vi "Build Shared Library Search Path.vi"(8 "Error In":errorcluster, 11 "labssh2 Shared Library":path=path "") -> (0 "Error Out":errorcluster, 3 "Search Path":path[](array[path])=[path "D:/Users/cfield/Code/Field R&D Services/SSH/LabSSH2/LabVIEW/trunk/src/LabSSH2/Private/labssh2.*"])   [LabVIEW 2017, in "Toolkit.lvlib"]
uses:
  Toolkit.lvlib
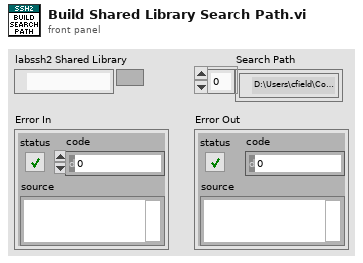
[diagram p1: front panel]
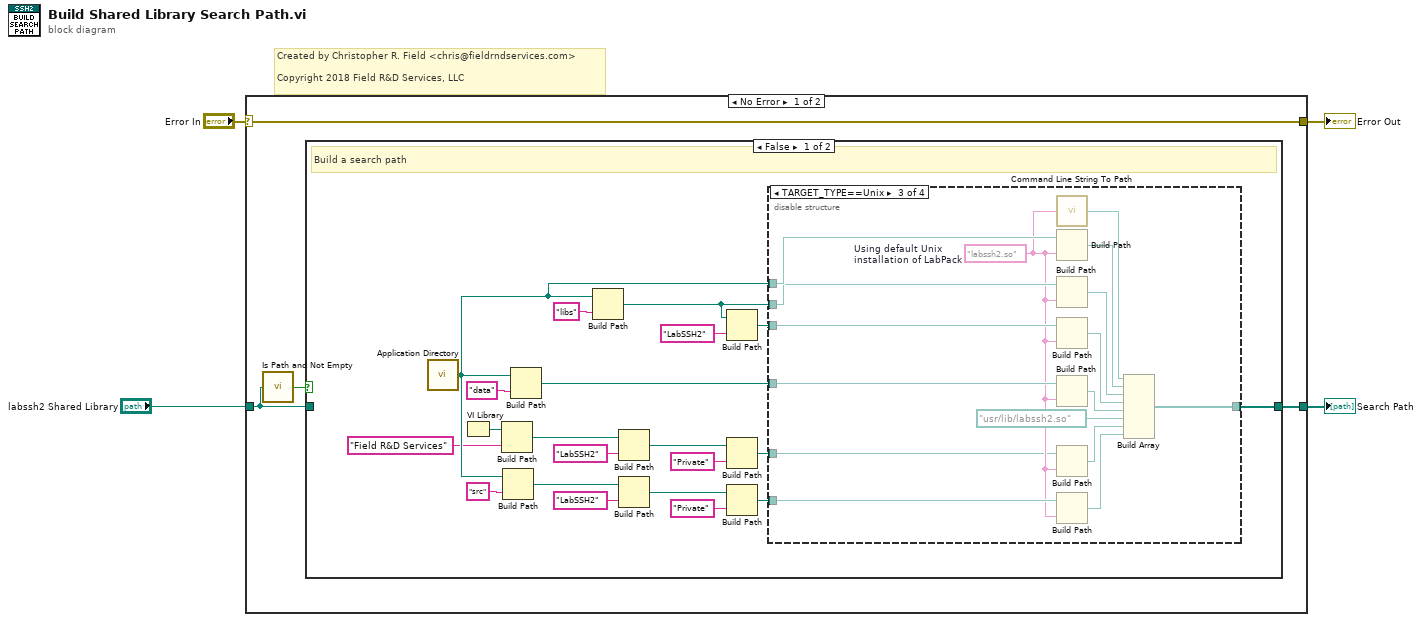
[diagram p0: block diagram]
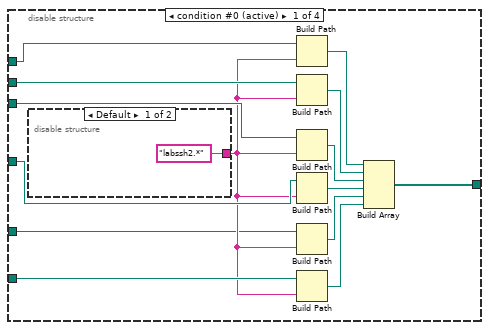
[diagram p2: hidden frame]
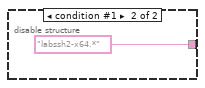
[diagram p3: hidden frame]
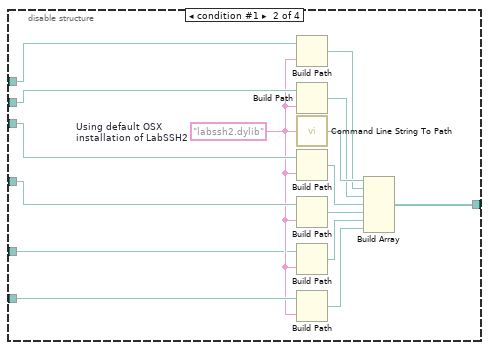
[diagram p4: hidden frame]
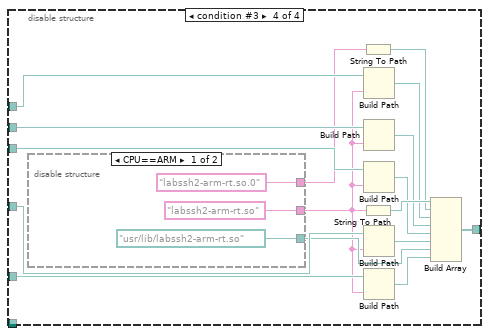
[diagram p5: hidden frame]
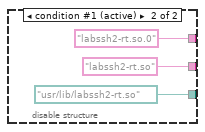
[diagram p6: hidden frame]
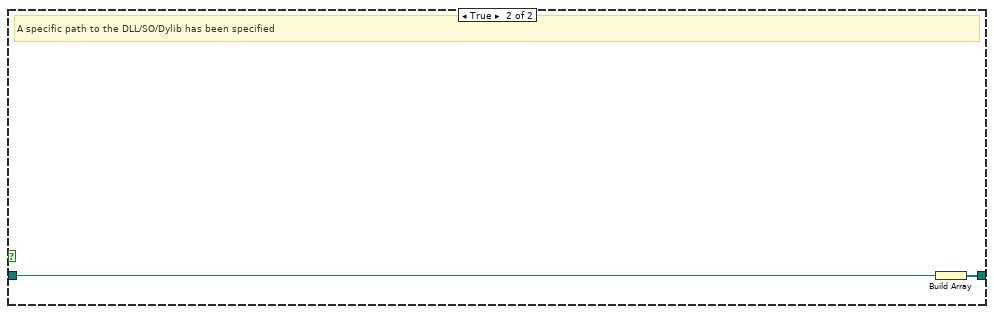
[diagram p7: hidden frame]
diagram:
  # "Created by Christopher R. Field <chris@fieldrndservices.com>\n\nCopyright 2018 Field R&D Services, LLC"
  n1 = case shown="No Error" "Error In" {
    selector: "Error In" -> [w5 w101]
    tunnel: [w8 _] -> w4
    tunnel: "labssh2 Shared Library" -> [w7 _]
    tunnel: [w5 w101] -> w1
    frame No Error {
      n2 = call <vilib>:"Is Path and Not Empty.vi"("path"=w7) -> ("Is Path and Not Empty?"=w6:bool)  [unwired: 4 in]
      n3 = case shown="False" w6 {
        tunnel: w7 -> [_ w100]
        tunnel: [w23 w99] -> w8
        frame False {
          # "Build a search path"
          n4 = call <vilib>:"Application Directory.vi"() -> ("Application Directory"=w21:path)
          n5 = VI Library() -> (path=w15:path)
          n6 = Build Path(base path=w15, name or relative path="Field R&D Services") -> (appended path=w13:path)
          n7 = Build Path ("EXE include\nlocation")(base path=w21, name or relative path="src") -> (appended path=w26:path)
          n8 = Build Path ("EXE include\nlocation")(base path=w21, name or relative path="data") -> (appended path=w19:path)
          n9 = Build Path ("EXE include\nlocation")(base path=w21, name or relative path="libs") -> (appended path=w18:path)
          n10 = Build Path(base path=w13, name or relative path="LabSSH2") -> (appended path=w11:path)
          n11 = Build Path ("EXE include\nlocation")(base path=w26, name or relative path="LabSSH2") -> (appended path=w28:path)
          n12 = Build Path ("EXE include\nlocation")(base path=w18, name or relative path="LabSSH2") -> (appended path=w16:path)
          n13 = Build Path(base path=w11, name or relative path="Private") -> (appended path=w9:path)
          n14 = Build Path ("EXE include\nlocation")(base path=w28, name or relative path="Private") -> (appended path=w24:path)
          n15 = disable-structure shown="TARGET_TYPE==Unix" {
            disable-tunnel: [w42 w59 w75 w92] -> w23
            disable-tunnel: w24 -> [w43 w58 w74 _]
            disable-tunnel: w21 -> [w41 w57 w68 w85]
            disable-tunnel: w18 -> [w40 w56 w67 w84]
            disable-tunnel: w19 -> [w39 w54 w65 w82]
            disable-tunnel: w16 -> [w38 w55 w66 w83]
            disable-tunnel: w9 -> [w36 w48 w63 w79]
            frame condition #0 (active) {
              n16 = disable-structure shown="Default" {
                disable-tunnel: ["labssh2.*" ("name or relative path") "labssh2-x64.*" ("name or relative path")] -> w37
                frame condition #0 (active) {
                }
                frame condition #1 {
                }
              }
              n17 = Build Path ("EXE include\nlocation")(base path=w41, name or relative path=w37) -> (appended path=w30:path)
              n18 = Build Path ("EXE include\nlocation")(base path=w40, name or relative path=w37) -> (appended path=w31:path)
              n19 = Build Path ("EXE include\nlocation")(base path=w38, name or relative path=w37) -> (appended path=w32:path)
              n20 = Build Path ("EXE include\nlocation")(base path=w39, name or relative path=w37) -> (appended path=w33:path)
              n21 = Build Path ("EXE include\nlocation")(base path=w36, name or relative path=w37) -> (appended path=w35:path)
              n22 = Build Path ("EXE include\nlocation")(base path=w43, name or relative path=w37) -> (appended path=w34:path)
              n23 = Build Array(w30, w31, w32, w33, w35, w34) -> (w42:path[])
            }
            frame condition #1 {
              w49 = "labssh2.dylib"  # Using default OSX installation of LabSSH2
              n24 = Build Path ("EXE include\nlocation")(base path=w57, name or relative path=w49) -> (appended path=w53:path)
              n25 = Build Path ("EXE include\nlocation")(base path=w56, name or relative path=w49) -> (appended path=w52:path)
              n26 = call <vilib>:"Command Line String To Path.vi"("string"=w49) -> ("path"=w60:path)
              n27 = Build Path ("EXE include\nlocation")(base path=w55, name or relative path=w49) -> (appended path=w51:path)
              n28 = Build Path ("EXE include\nlocation")(base path=w54, name or relative path=w49) -> (appended path=w50:path)
              n29 = Build Path ("EXE include\nlocation")(base path=w48, name or relative path=w49) -> (appended path=w47:path)
              n30 = Build Path ("EXE include\nlocation")(base path=w58, name or relative path=w49) -> (appended path=w46:path)
              n31 = Build Array(w60, w53, w52, w51, w50, w47, w46) -> (w59:path[])
            }
            frame condition #2 {
              w64 = "labssh2.so"  # Using default Unix installation of LabPack
              n32 = call <vilib>:"Command Line String To Path.vi"("string"=w64) -> ("path"=w76:path)
              n33 = Build Path ("EXE include\nlocation")(base path=w68, name or relative path=w64) -> (appended path=w72:path)
              n34 = Build Path ("EXE include\nlocation")(base path=w67, name or relative path=w64) -> (appended path=w71:path)
              n35 = Build Path ("EXE include\nlocation")(base path=w66, name or relative path=w64) -> (appended path=w70:path)
              n36 = Build Path ("EXE include\nlocation")(base path=w65, name or relative path=w64) -> (appended path=w69:path)
              n37 = Build Path ("EXE include\nlocation")(base path=w63, name or relative path=w64) -> (appended path=w62:path)
              n38 = Build Path ("EXE include\nlocation")(base path=w74, name or relative path=w64) -> (appended path=w61:path)
              n39 = Build Array(w76, w72, w71, w70, w69, path "/usr/lib/labssh2.so" ("path"), w62, w61) -> (w75:path[])
            }
            frame condition #3 {
              n40 = disable-structure shown="CPU==ARM" {
                disable-tunnel: ["labssh2-arm-rt.so.0" "labssh2-rt.so.0"] -> w81
                disable-tunnel: ["labssh2-arm-rt.so" "labssh2-rt.so"] -> w78
                disable-tunnel: [path "/usr/lib/labssh2-arm-rt.so" ("path") path "/usr/lib/labssh2-rt.so" ("path")] -> w80
                frame condition #0 {
                }
                frame condition #1 (active) {
                }
              }
              n41 = String To Path(string=w81) -> (path=w90:path)
              n42 = String To Path(string=w78) -> (path=w91:path)
              n43 = Build Path ("EXE include\nlocation")(base path=w85, name or relative path=w78) -> (appended path=w86:path)
              n44 = Build Path ("EXE include\nlocation")(base path=w84, name or relative path=w78) -> (appended path=w89:path)
              n45 = Build Path ("EXE include\nlocation")(base path=w83, name or relative path=w78) -> (appended path=w88:path)
              n46 = Build Path ("EXE include\nlocation")(base path=w82, name or relative path=w78) -> (appended path=w87:path)
              n47 = Build Path ("EXE include\nlocation")(base path=w79, name or relative path=w78) -> (appended path=w77:path)
              n48 = Build Array(w91, w90, w86, w89, w88, w87, w80, w77) -> (w92:path[])
            }
          }
        }
        frame True {
          # "A specific path to the DLL/SO/Dylib has been specified"
          n49 = Build Array(w100) -> (w99:path[])
        }
      }
    }
    frame Error {
    }
  }
  "Search Path" <- w4
  "Error Out" <- w1
